vi "Fill Factor.vi"(8 "Current at Short Circuit":dbl, 9 "Voltage at Open Circuit":dbl, 10 "Voltage at Max Power":dbl, 11 "Current at Max Power":dbl) -> (3 "Fill factor":dbl)   [LabVIEW 2016]
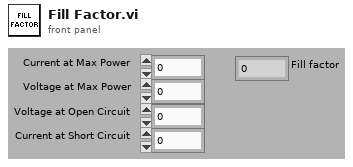
[diagram p1: front panel]
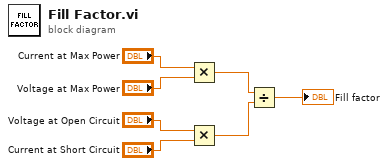
[diagram p0: block diagram]
diagram:
  n1 = Multiply(x="Current at Max Power", y="Voltage at Max Power") -> (x*y=w3:dbl)
  n2 = Multiply(x="Voltage at Open Circuit", y="Current at Short Circuit") -> (x*y=w2:dbl)
  n3 = Divide(x=w3, y=w2) -> (x/y=→"Fill factor":dbl)
